vi "PicoScope5000aWrapSettings.vi"(1 "enabled array":i16[](array[numeric]), 8 "Device Info":T1, 10 "Handle In":i16, 11 "error in (no error)":errorcluster) -> (2 "Handle Out":i16, 3 "error out":errorcluster)   [LabVIEW 2010]
uses:
  ps5000a.dll
  ps5000aWrap.dll
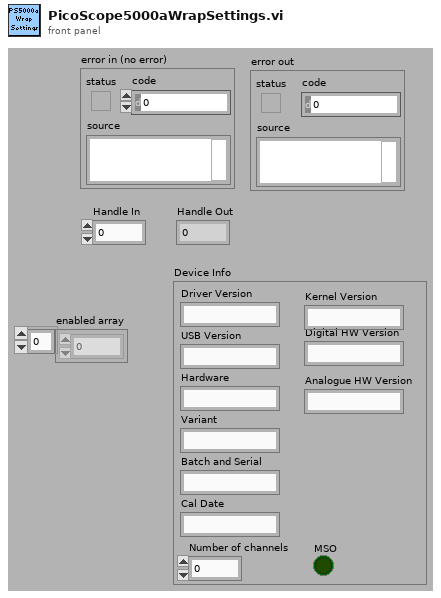
[diagram p1: front panel]
types:
  T1 = cluster{"Driver Version":string, "USB Version":string, "Hardware":string, "Variant":string, "Batch and Serial":string, "Cal Date":string, "Kernel Version":string, "Digital HW Version":string, "Analogue HW Version":string, "MSO":bool, "Number of channels":i16}
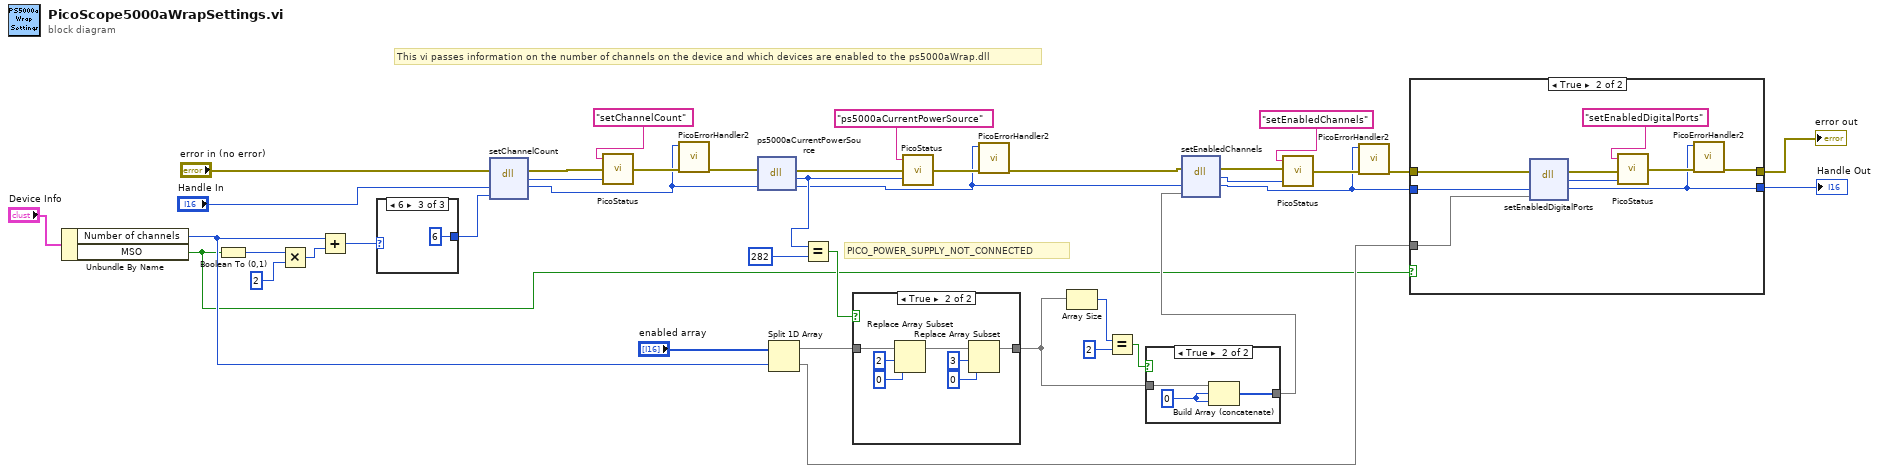
[diagram p0: block diagram]
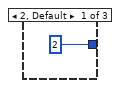
[diagram p5: hidden frame]
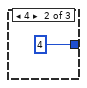
[diagram p6: hidden frame]
diagram:
  # "PICO_POWER_SUPPLY_NOT_CONNECTED"
  # "This vi passes information on the number of channels on the device and which devices are enabled to the ps5000aWrap.dll"
  n1 = Unbundle By Name("Device Info") -> ("Number of channels"=w7:i16, "MSO"=w1:bool)
  n2 = Boolean To (0,1)(Boolean=w1) -> (0, 1=w34:i16)
  n3 = Multiply(x=w34, y=i16 2) -> (x*y=w32:i16)
  n4 = Add(x=w7, y=w32) -> (x+y=w35:i16)
  n5 = case shown="6" w35 {
    tunnel: [i16 2 i16 4 i16 6] -> w38
    frame 2, Default {
    }
    frame 4 {
    }
    frame 6 {
    }
  }
  n6 = dll-call lib="ps5000aWrap.dll" fn="setChannelCount"(error in="error in (no error)", "handle"="Handle In", "channelCount"=w38) -> (error out=w17:errorcluster, "PICO_STATUS"=w14:u32, "handle"=w13:i16)  [unwired: 3 in, 1 out]
  n7 = call "PicoStatus.vi"("PICO STATUS"=w14, "error in"=w17, "source"="setChannelCount") -> ("error out"=w19:errorcluster)
  n8 = call "PicoErrorHandler2.vi"("error in (no error)"=w19, "handle In"=w13) -> ("error out"=w15:errorcluster)  [unwired: 9 in]
  n9 = dll-call lib="ps5000a.dll" fn="ps5000aCurrentPowerSource"(error in=w15, "handle"=w13) -> (error out=w30:errorcluster, "PICO STATUS"=w21:u32, "handle"=w20:i16)  [unwired: 2 in, 1 out]
  n10 = Split 1D Array(array="enabled array", index=w7) -> (first subarray=w23:i16[], second subarray=w25:i16[])
  n11 = Equal?(x=w21, y=u32 282) -> (x = y?=w22:bool)
  n12 = case shown="True" w22 {
    tunnel: [w44 w50] -> w3
    tunnel: w23 -> [w44 w49]
    frame False {
    }
    frame True {
      n13 = Replace Array Subset(array=w49, new element=i16 0 ("new element/subarray"), index=2) -> (w51:i16[])
      n14 = Replace Array Subset(array=w51, new element=i16 0 ("new element/subarray"), index=3) -> (w50:i16[])
    }
  }
  n15 = call "PicoStatus.vi"("PICO STATUS"=w21, "error in"=w30, "source"="ps5000aCurrentPowerSource") -> ("error out"=w29:errorcluster)
  n16 = call "PicoErrorHandler2.vi"("error in (no error)"=w29, "handle In"=w20) -> ("error out"=w28:errorcluster)  [unwired: 9 in]
  n17 = Array Size(array=w3) -> (size(s)=w4:i32)
  n18 = Equal?(x=w4, y=2) -> (x = y?=w5:bool)
  n19 = case shown="True" w5 {
    tunnel: w3 -> [w52 w55]
    tunnel: [w52 w53] -> w2
    frame False {
    }
    frame True {
      w54 = i16 0 ("y")
      n20 = Build Array (concatenate)(w55, w54, w54) -> (w53:i16[])
    }
  }
  n21 = dll-call lib="ps5000aWrap.dll" fn="setEnabledChannels"(error in=w28, "handle"=w20, "enabledChannels"=w2) -> (error out=w12:errorcluster, "PICO_STATUS"=w10:u32, "handle"=w8:i16)  [unwired: 3 in, 1 out]
  n22 = call "PicoStatus.vi"("PICO STATUS"=w10, "error in"=w12, "source"="setEnabledChannels") -> ("error out"=w18:errorcluster)
  n23 = call "PicoErrorHandler2.vi"("error in (no error)"=w18, "handle In"=w8) -> ("error out"=w9:errorcluster)  [unwired: 9 in]
  n24 = case shown="True" w1 {
    tunnel: w9 -> [w57 w66]
    tunnel: w8 -> [w56 w65]
    tunnel: [w57 w59] -> w27
    tunnel: [w56 w58] -> w26
    tunnel: w25 -> [_ w64]
    frame False {
    }
    frame True {
      n25 = dll-call lib="ps5000aWrap.dll" fn="setEnabledDigitalPorts"(error in=w66, "handle"=w65, "enabledChannels"=w64) -> (error out=w62:errorcluster, "PICO_STATUS"=w60:u32, "handle"=w58:i16)  [unwired: 3 in, 1 out]
      n26 = call "PicoStatus.vi"("PICO STATUS"=w60, "error in"=w62, "source"="setEnabledDigitalPorts") -> ("error out"=w63:errorcluster)
      n27 = call "PicoErrorHandler2.vi"("error in (no error)"=w63, "handle In"=w58) -> ("error out"=w59:errorcluster)  [unwired: 9 in]
    }
  }
  "Handle Out" <- w26
  "error out" <- w27
